vi "dialog save dirty dot.vi"(8 "error in":errorcluster, 9 "View":refnum<vi>, 10 "sub panel ref in":refnum<vi>, 11 "state in":T1) -> (0 "error out":errorcluster, 1 "new":bool, 3 "state out":T1)   [LabVIEW 2013, in "configuration library.lvlib"]
uses:
  configuration library.lvlib
  Controls/StateCluster.ctl
  <vilib>/NI/Configuration Framework/Node/NodeRef.ctl
  <vilib>/NI/Configuration Framework/Node/NISE_CEF_Node.lvclass
  <vilib>/NI/Configuration Framework/Node/UserEventRef.ctl
  <vilib>/NI/Configuration Framework/Controls/EventCluster.ctl
  <vilib>/NI/Configuration Framework/NISE_CEF_TreeControl.lvlib
  SplashScreen/notifier data.ctl
  SplashScreen/splash screen.lvlib
  SplashScreen/splash screen.ctl
  <vilib>/NI/Tag Bus Data Framework/Configuration Editor/Classes/SystemConfigRepo/SystemConfigRepo.lvclass
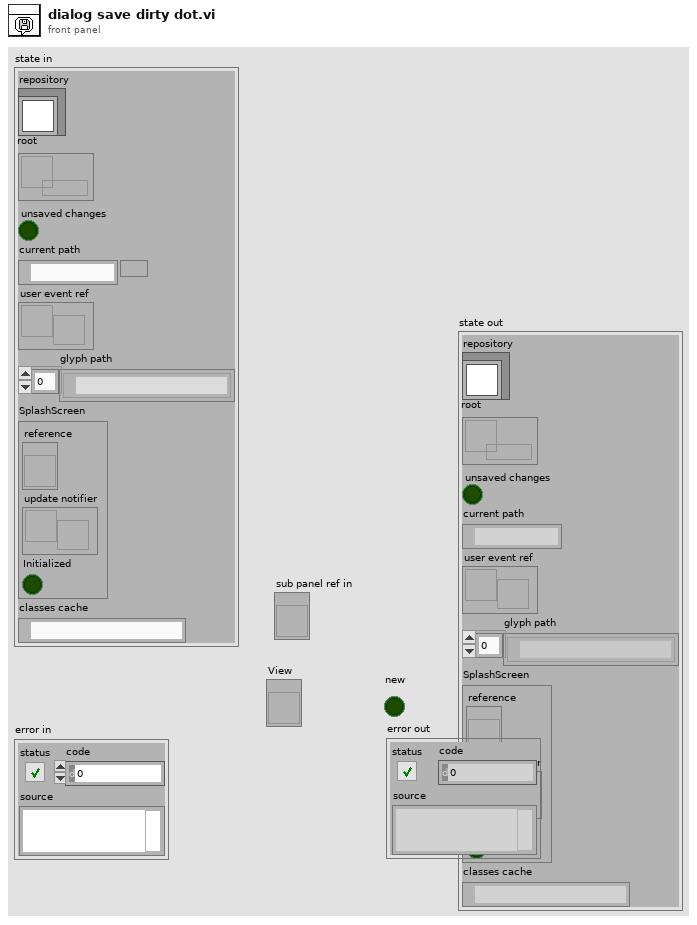
[diagram p1: front panel]
types:
  T1 = typedef "configuration library.lvlib/StateCluster.ctl" = cluster{"repository":refnum<class "SystemConfigRepo.lvclass">, "root":T2, "unsaved changes":bool, "current path":path, "user event ref":T3, "glyph path":path[], "SplashScreen":T4, "classes cache":path}
  T2 = typedef "NISE_CEF_Node.lvclass/NodeRef.ctl" = refnum<data-value>
  T3 = typedef "NISE_CEF_Node.lvclass/UserEventRef.ctl" = refnum<user-event>
  T4 = typedef "configuration library.lvlib/splash screen.lvlib/splash screen.ctl" = cluster{"reference":refnum<vi>, "update notifier":refnum<notifier>, "Initialized":bool}
  T5 = enum16{"Left Button", "Center Button", "Right Button", "Window Close"}
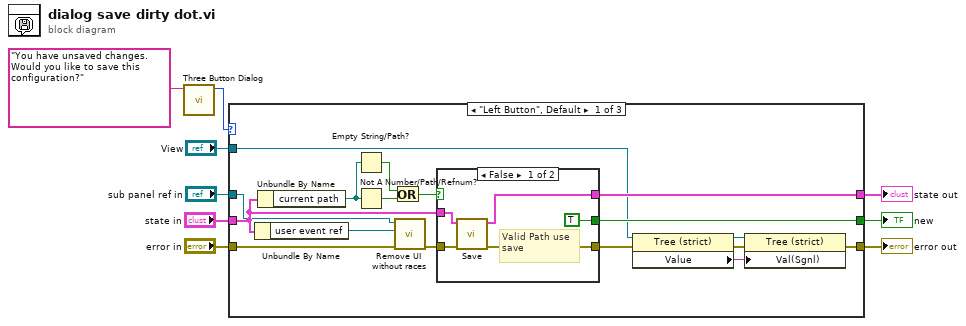
[diagram p0: block diagram]
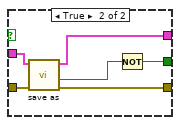
[diagram p2: hidden frame]
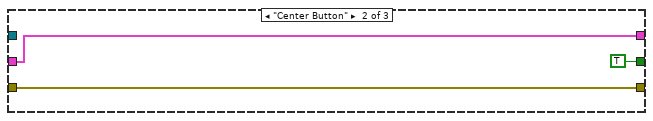
[diagram p3: hidden frame]
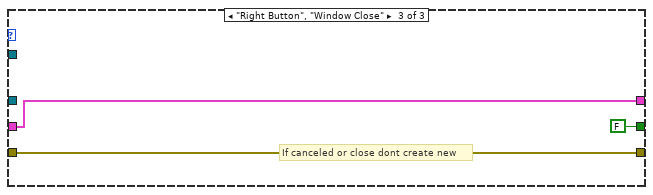
[diagram p4: hidden frame]
diagram:
  n1 = call <vilib>:"Three Button Dialog.vi"("message"="You have unsaved changes.  Would you like to save this configuration?") -> ("Which Button?"=w4:T5)  [unwired: 10 in]
  n2 = case shown="\"Left Button\", Default" w4 {
    tunnel: "state in" -> [w20 w39 w42]
    tunnel: [w22 w39 w42] -> w8
    tunnel: "error in" -> [w19 w38 w41]
    tunnel: [w12 w38 w41] -> w6
    tunnel: [w21 TRUE ("New") FALSE ("New")] -> w3
    tunnel: "sub panel ref in" -> [w17 _ _]
    tunnel: "View" -> [w11 _ _]
    frame "Left Button", Default {
      n3 = Unbundle By Name(w20) -> ("user event ref"=w16:T3)
      n4 = Unbundle By Name(w20) -> ("current path"=w26:path)
      n5 = Empty String/Path?(string/path=w26) -> (empty?=w24:bool)
      n6 = Not A Number/Path/Refnum?(number/path/refnum=w26) -> (NaN/Path/Refnum?=w23:bool)
      n7 = Or(x=w24, y=w23) -> (x .or. y?=w25:bool)
      n8 = call "Remove UI without races.vi"("error in"=w19, "user event ref"=w16, "sub panel ref in"=w17) -> ("error out"=w18:errorcluster)  [unwired: 7 in, 1 out]
      n9 = case shown="False" w25 {
        tunnel: w20 -> [w28 w35]
        tunnel: [w31 w34] -> w22
        tunnel: [w27 w36] -> w13
        tunnel: w18 -> [w29 w37]
        tunnel: [TRUE w32] -> w21
        frame False {
          # "Valid Path use save"
          n10 = call "Save.vi"("error in"=w29, "state in"=w28) -> ("error out"=w27:errorcluster, "state out"=w31:T1)  [unwired: 8 in]
        }
        frame True {
          n11 = call "save as.vi"("error in"=w37, "state in"=w35) -> ("error out"=w36:errorcluster, "canceled?"=w33:bool, "state out"=w34:T1)  [unwired: 7 in]
          n12 = Not(x=w33) -> (.not. x?=w32:bool)
        }
      }
      n13 = property class="Tree (strict)"(reference=w11, error in=w13) -> (reference out=w10:refnum<vi>, error out=w15:errorcluster, "Value"=w14:string)
      n14 = property class="Tree (strict)"(reference=w10, error in=w15, "Val(Sgnl)"=w14) -> (error out=w12:errorcluster)  [unwired: 1 out]
    }
    frame "Center Button" {
    }
    frame "Right Button", "Window Close" {
      # "If canceled or close dont create new"
    }
  }
  "state out" <- w8
  "error out" <- w6
  "new" <- w3
